vi "Global 1.vi"() -> ()   [LabVIEW 2017]
panel:
  out "back to inipos":bool
  out "LA Auto/cal":bool
  out "Shot - Act/pas":bool
  out "LA position":i32
  out "Trigger rod":string
  out "Shot detector":string
  out "From Python":string
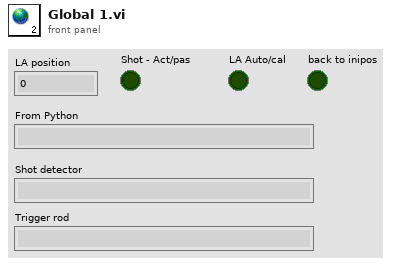
[diagram p1: front panel]
diagram:
